vi "Save EventLog.vi"(8 "Error In":errorcluster, 11 "EventLog in":refnum<class "EventLog.lvclass">) -> (0 "Error Out":errorcluster, 3 "EventLog out":refnum<class "EventLog.lvclass">)   [LabVIEW 2019, in "EventLog.lvlib" / "EventLog.lvclass"]
uses:
  EventLog.lvclass
  C:/Projekty/_Poboczne/PC_ActorFramework/07_Program/LABVIEW/02_Source/SubModules/LogsAbstract/LogsAbstract.lvclass
  EventLog.lvclass/EventLog.ctl
  Classes/Events/Events.lvclass/Events.ctl
  LogsAbstract/LogsAbstract.lvclass/LogsAbstract.ctl
  8ebcb51d-6aa0-4ebd-80a8-675e538a3599.vi
  8ebcb51d-6aa0-4ebd-80a8-675e538a3599.vi/3945156b-860f-474e-959e-68229f997543.vi
  LogsAbstract/Accessors/Write LogPath.vi
  LogsAbstract/Accessors/Read LogPath.vi
  <vilib>/Utility/file.llb/Write Delimited Spreadsheet.vi
  <vilib>/Utility/file.llb/Write Delimited Spreadsheet (string).vi
  Classes/Events/Events.lvclass
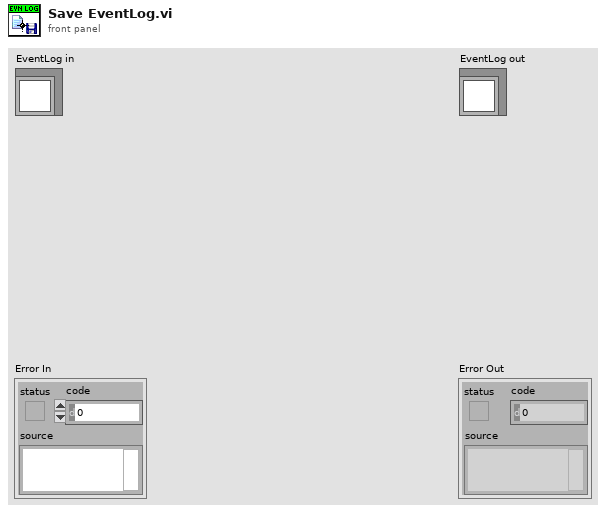
[diagram p1: front panel]
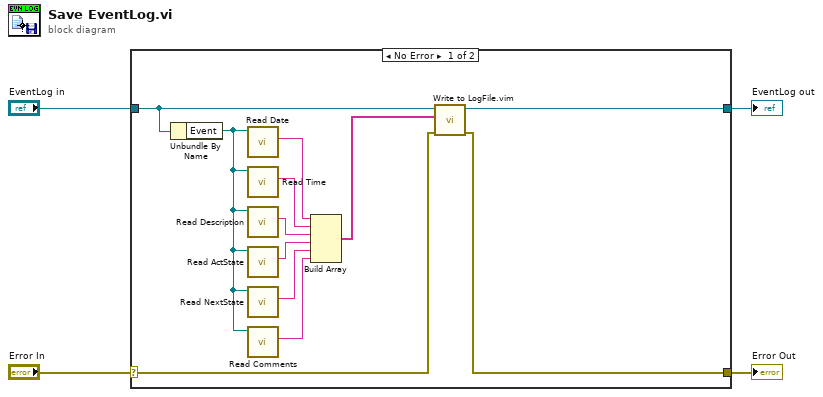
[diagram p0: block diagram]
diagram:
  n1 = case shown="No Error" "Error In" {
    selector: "Error In" -> [w6 w18]
    tunnel: [w5 w18] -> w3
    tunnel: [w15 w17] -> w1
    tunnel: "EventLog in" -> [w16 w17]
    frame No Error {
      n2 = Unbundle By Name(w16) -> ("Event"=w14:refnum<class "Events.lvclass">)
      n3 = call "Read Date.vi"("Events in"=w14) -> ("Date"=w8:string)  [unwired: 8 in, 2 out]
      n4 = call "Read Time.vi"("Events in"=w14) -> ("Time"=w11:string)  [unwired: 8 in, 2 out]
      n5 = call "Read Description.vi"("Events in"=w14) -> ("Description"=w12:string)  [unwired: 8 in, 2 out]
      n6 = call "Read ActState.vi"("Events in"=w14) -> ("ActState"=w13:string)  [unwired: 8 in, 2 out]
      n7 = call "Read NextState.vi"("Events in"=w14) -> ("NexttState"=w10:string)  [unwired: 8 in, 2 out]
      n8 = call "Read Comments.vi"("Events in"=w14) -> ("Comments"=w9:string)  [unwired: 8 in, 2 out]
      n9 = Build Array(w8, w11, w12, w13, w10, w9) -> (w7:string[])
      n10 = call "Write to LogFile.vim"("Error In"=w6, "Data"=w7, "LogClass In"=w16) -> ("Error out"=w5:errorcluster, "LogClass Out"=w15:refnum<class "EventLog.lvclass">)  [unwired: 7 in]
    }
    frame Error {
    }
  }
  "Error Out" <- w3
  "EventLog out" <- w1
